vi "Server FGV.vi"(7 "Mode":T10(ring), 8 "error in":errorcluster, 10 "New Server":T1 caption="Server", 11 "id":i32) -> (0 "error out":errorcluster, 1 "server reference":refnum<data-value>, 2 "new id":i32, 4 "all servers":refnum<data-value>[](array[refnum]), 6 "server ids":i32[](array[numeric]))   [LabVIEW 2025, in "MCP Server.lvlib"]
doc: "Stores and retrieves the DVRs to individual server instances. Uses a variant lookup table internally."
uses:
  MCP Server.lvlib
  Server Data.ctl
  <vilib>/IlluminatedG/IG HTTP Server/HTTP Server/Server/Server.lvclass
  Tool Data.ctl
  Input Parameter.ctl
  Output Parameter.ctl
  Logging.ctl
  User Events.ctl
  onRpc.ctl
  Prompt Data.ctl
  Prompt Argument.ctl
  resource data.ctl
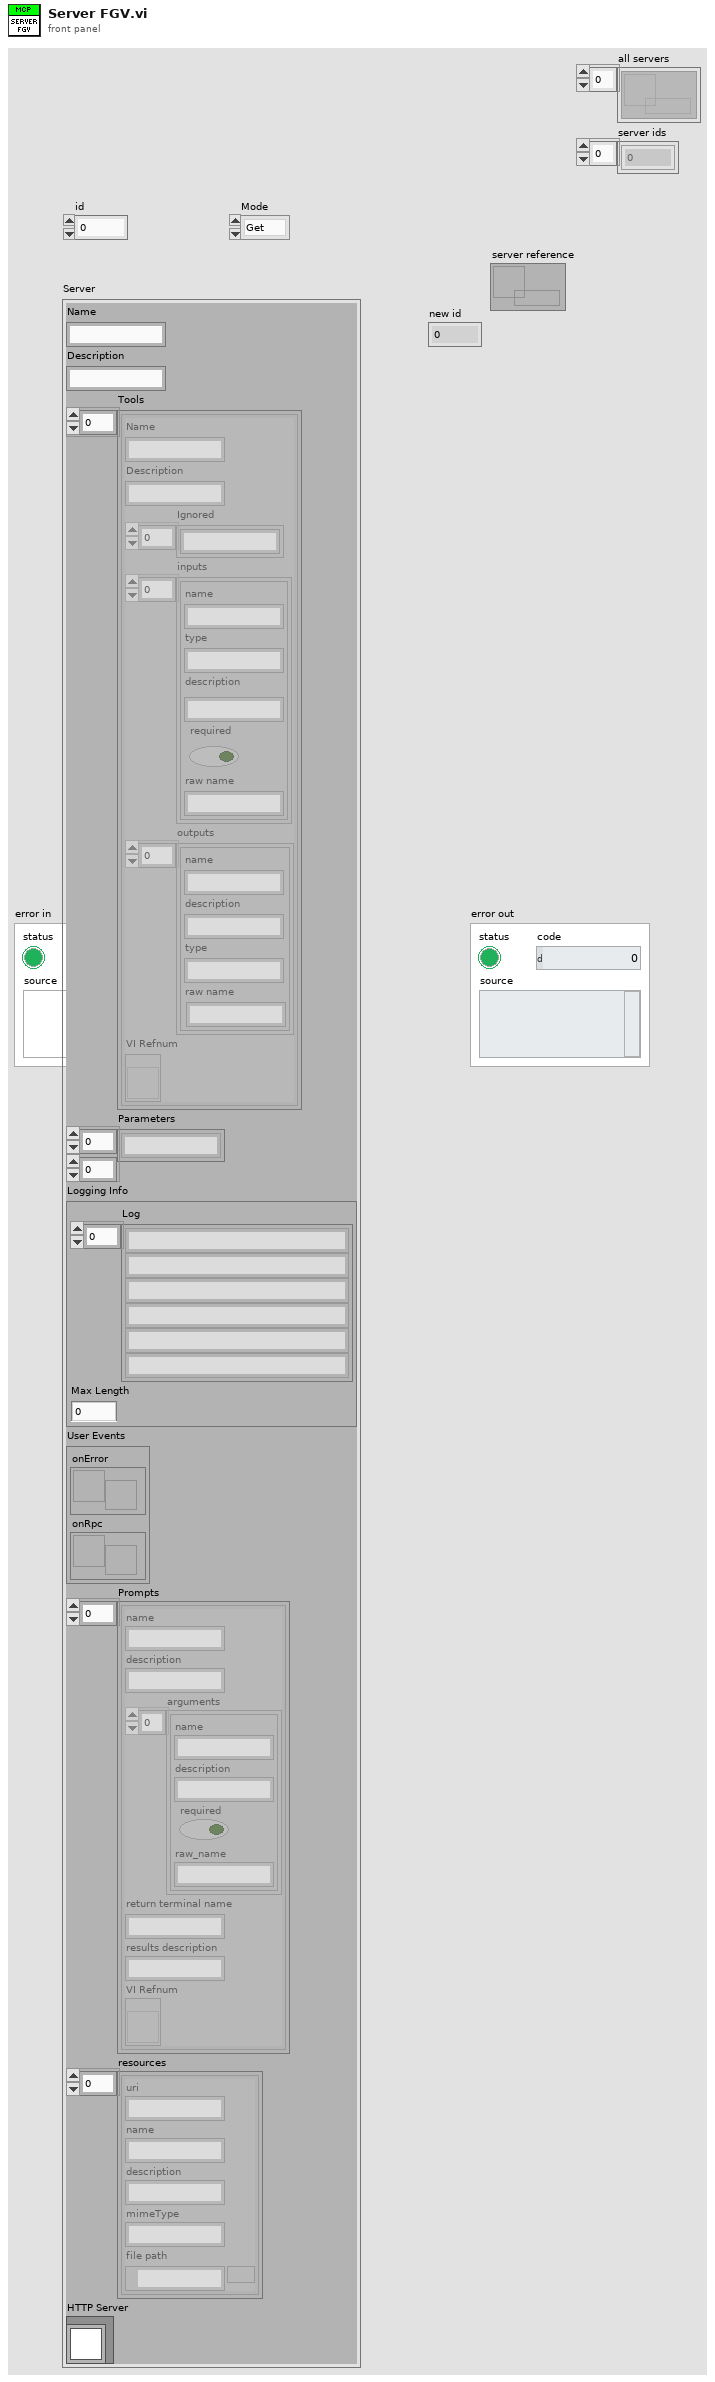
[diagram p1: front panel]
types:
  T1 = typedef "MCP Server.lvlib/Server Data.ctl" = cluster{"Name":string, "Description":string, "Tools":T2[], "Parameters":string[][], "Logging Info":T5, "User Events":T6, "Prompts":T7[], "resources":T9[], "HTTP Server":refnum<class "Server.lvclass">}
  T2 = typedef "MCP Server.lvlib/Tool Data.ctl" = cluster{"Name":string, "Description":string, "Ignored":string[], "inputs":T3[], "outputs":T4[], "VI Refnum":refnum<vi>}
  T3 = typedef "MCP Server.lvlib/Input Parameter.ctl" = cluster{"name":string, "type":string, "description":string, "required":bool, "raw name":string}
  T4 = typedef "MCP Server.lvlib/Output Parameter.ctl" = cluster{"name":string, "description":string, "type":string, "raw name":string}
  T5 = typedef "MCP Server.lvlib/Logging.ctl" = cluster{"Log":string[], "Max Length":i32}
  T6 = typedef "MCP Server.lvlib/User Events.ctl" = cluster{"onError":refnum<user-event>, "onRpc":refnum<user-event>}
  T7 = typedef "MCP Server.lvlib/Prompt Data.ctl" = cluster{"name":string, "description":string, "arguments":T8[], "return terminal name":string, "results description":string, "VI Refnum":refnum<vi>}
  T8 = typedef "MCP Server.lvlib/Prompt Argument.ctl" = cluster{"name":string, "description":string, "required":bool, "raw_name":string}
  T9 = typedef "MCP Server.lvlib/resource data.ctl" = cluster{"uri":string, "name":string, "description":string, "mimeType":string, "file path":path}
  T10 = enum16{"Get", "GetAll", "Add", "Remove", "Clear"}
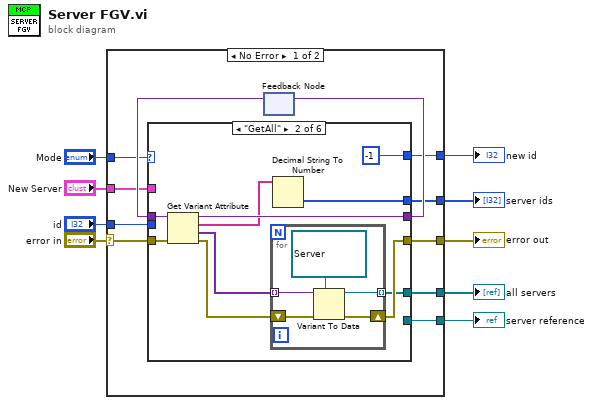
[diagram p0: block diagram]
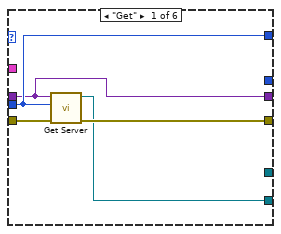
[diagram p2: hidden frame]
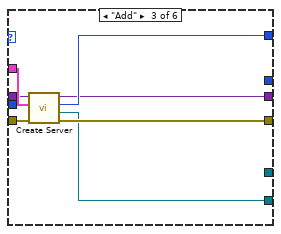
[diagram p3: hidden frame]
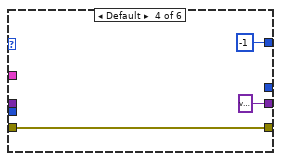
[diagram p4: hidden frame]
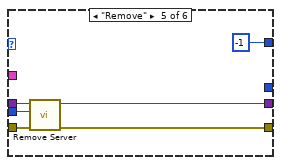
[diagram p5: hidden frame]
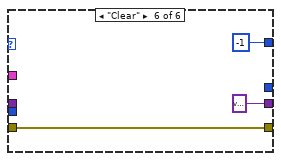
[diagram p6: hidden frame]
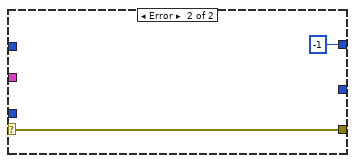
[diagram p7: hidden frame]
diagram:
  n1 = case shown="No Error" "error in" {
    selector: "error in" -> [w13 w62]
    tunnel: "Mode" -> [w18 _]
    tunnel: "id" -> [w17 _]
    tunnel: [w10 -1 ("id")] -> w7
    tunnel: [w16 w62] -> w6
    tunnel: [w15 _] -> w5
    tunnel: "New Server" -> [w14 _]
    tunnel: [w12 _] -> w2
    tunnel: [w11 _] -> w1
    frame No Error {
      n2 = feedback #1() -> (w19:variant)  [unwired: 1 in]
      n3 = case shown="\"GetAll\"" w18 {
        tunnel: [w21 w34 w41 variant w57 variant] -> w20
        tunnel: w19 -> [w21 w35 w44 _ w54 _]
        tunnel: w17 -> [w22 _ w45 _ w53 _]
        tunnel: w13 -> [w25 w33 w47 w50 w56 w60]
        tunnel: [w24 w30 w46 w50 w55 w60] -> w16
        tunnel: [w23 _ w42 _ _ _] -> w15
        tunnel: w14 -> [_ _ w48 _ _ _]
        tunnel: [_ w29 _ _ _ _] -> w12
        tunnel: [_ w27 _ _ _ _] -> w11
        tunnel: [w22 -1 ("id") w43 -1 -1 -1] -> w10
        frame "Get" {
          n4 = call "Get Server.vi"("error in (no error)"=w25, "id"=w22, "Variant in"=w21) -> ("error out"=w24:errorcluster, "Data Value Reference out"=w23:refnum<data-value>)  [unwired: 7 in]
        }
        frame "GetAll" {
          n5 = Get Variant Attribute(Variant=w35, error in=w33) -> (duplicate Variant=w34:variant, names=w28:string[], values=w32:variant[], error out=w31:errorcluster)  [unwired: 2 in]
          n6 = for {
            tunnel: w32 -> [w40] mode=indexing
            shift-right: [w38] -> w30
            shift-left: w31 -> [w39]
            tunnel: [w36] -> w29 mode=indexing
            n7 = Variant To Data(error in=w39, type=refnum<data-value> refnum ("data value reference"), Variant=w40) -> (data=w36:refnum<data-value>, error out=w38:errorcluster)
          }
          n8 = Decimal String To Number(string=w28) -> (number=w27:i32[])  [unwired: 2 in, 1 out]
        }
        frame "Add" {
          n9 = call "Create Server.vi"("error in (no error)"=w47, "id"=w45, "New Server"=w48, "Variant in"=w44) -> ("error out"=w46:errorcluster, "Data Value Reference out"=w42:refnum<data-value>, "unique server id out"=w43:i32, "Variant"=w41:variant)  [unwired: 4 in]
        }
        frame Default {
        }
        frame "Remove" {
          n10 = call "Remove Server.vi"("error in (no error)"=w56, "id"=w53, "Variant in"=w54) -> ("error out"=w55:errorcluster, "Variant out"=w57:variant)  [unwired: 7 in]
        }
        frame "Clear" {
        }
      }
      n11 = feedback-in #1(w20) -> ()
    }
    frame Error {
    }
  }
  "error out" <- w6
  "new id" <- w7
  "server reference" <- w5
  "all servers" <- w2
  "server ids" <- w1
